vi "Change Output DT.vi"(6 "Variant":variant, 8 "error in (no error)":errorcluster, 9 "old values":string[][](array[string]), 10 "object ref in":T2, 11 "Cluster":T3) -> (0 "error out":errorcluster)   [LabVIEW 2013, in "Scaling editor node.lvclass"]
uses:
  Scaling editor node.lvclass
  <vilib>/NI/DCAF Table API/Table Manager/Cell Change.ctl
  <vilib>/NI/DCAF Table API/Table Manager/object ref.ctl
  <vilib>/NI/DCAF/Tag Editor Core/Configuration Editor/Classes/Engine Parent/Engine Parent Editor Node.lvclass
  <vilib>/NI/DCAF/Tag Editor Core/Configuration Editor/Classes/Module editor node/module editor node.lvclass
  module/configuration/controls/scale data types.ctl
  module/configuration/Scaling configuration.lvclass
  Scaling editor node.lvclass/Scaling editor node.ctl
  <vilib>/NI/DCAF Table API/Table Manager.lvlib
  <vilib>/NI/DCAF Table API/Table Manager/Table Manager.lvclass
panel:
  in  "dt":T1
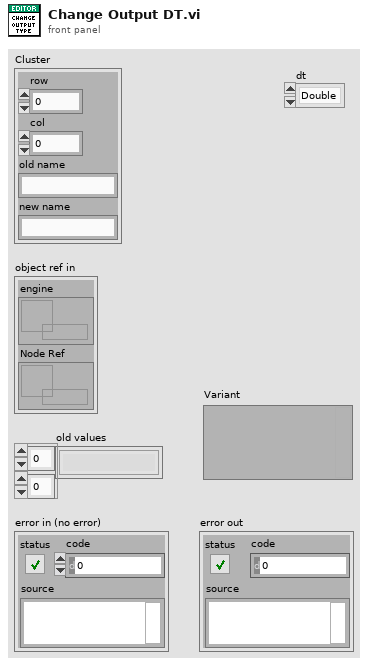
[diagram p1: front panel]
types:
  T1 = typedef "Scaling configuration.lvclass/scale data types.ctl" = enum16{"Double", "Single", "I64", "I32", "I16", "I8", "U64", "U32", "U16", "U8", "Boolean (0,1)"}
  T2 = typedef "Table Manager.lvlib/Table Manager.lvclass/object ref.ctl" = cluster{"engine":refnum<data-value>, "Node Ref":refnum<data-value>}
  T3 = typedef "Table Manager.lvlib/Cell Change.ctl" = cluster{"row":i32, "col":i32, "old name":string, "new name":string}
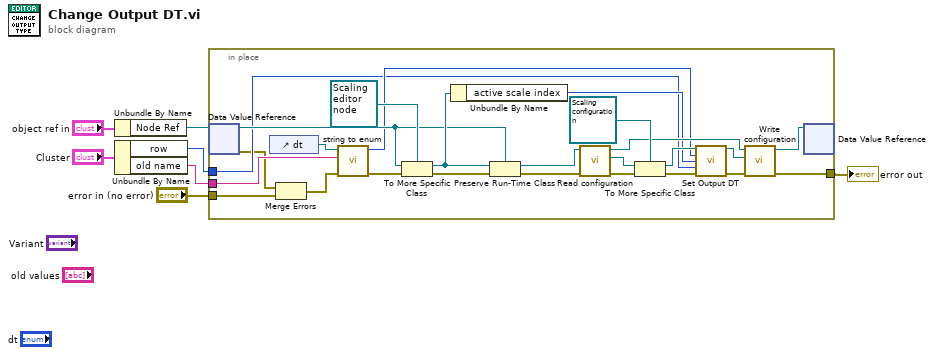
[diagram p0: block diagram]
diagram:
  n1 = Unbundle By Name("object ref in") -> ("Node Ref"=w3:refnum<data-value>)
  n2 = Unbundle By Name("Cluster") -> ("row"=w5:i32, "old name"=w2:string)
  n3 = in-place {
    in-place-border: w5 -> [w11]
    in-place-border: [w23] -> w1
    in-place-border: w2 -> [w14]
    in-place-border: "error in (no error)" -> [w9]
    n4 = in-place-dvr #1(w3) -> (w22:refnum<class "module editor node.lvclass">, w10:errorcluster)
    n5 = control-ref of="dt"() -> (w15:refnum<vi>)
    n6 = Merge Errors(w10, w9) -> (w8:errorcluster)
    n7 = call <vilib>:"string to enum.vi"("error in"=w8, "String"=w14, "Enum"=w15) -> ("error out"=w16:errorcluster, "Value"=w13:i32)  [unwired: 7 in]
    n8 = To More Specific Class(target class=refnum<class "Scaling editor node.lvclass"> refnum ("Scaling editor node"), reference=w22, error in=w16) -> (specific class reference=w28:refnum<class "Scaling editor node.lvclass">, error out=w21:errorcluster)
    n9 = Unbundle By Name(w28) -> ("active scale index"=w12:i32)
    n10 = Preserve Run-Time Class(object in=w28, error in=w21, 2:w22) -> (object out=w27:refnum<class "module editor node.lvclass">, error out=w26:errorcluster)
    n11 = call-dynamic "Read configuration.vi"("error in"=w26, "NISE_CEF_serializable node in"=w27) -> ("error out"=w25:errorcluster, "configuration"=w30:refnum<class "NISE_CEF_serializable configuration.lvclass">, "NISE_CEF_serializable node out"=w24:refnum<class "module editor node.lvclass">)  [unwired: 7 in]
    n12 = To More Specific Class(target class=refnum<class "Scaling configuration.lvclass"> refnum ("Scaling configuration"), reference=w30, error in=w25) -> (specific class reference=w17:refnum<class "Scaling configuration.lvclass">, error out=w18:errorcluster)
    n13 = call "Set Output DT.vi"("Scaling configuration in"=w17, "Scale Data Type"=w13, "Scale Index"=w12, "Mapping Index"=w11, "error in (no error)"=w18) -> ("Scaling configuration out"=w20:refnum<class "Scaling configuration.lvclass">, "error out"=w19:errorcluster)  [unwired: 9 in]
    n14 = call-dynamic "Write configuration.vi"("error in"=w19, "configuration"=w20, "NISE_CEF_serializable node in"=w24) -> ("error out"=w23:errorcluster, "NISE_CEF_serializable node out"=w32:refnum<class "module editor node.lvclass">)  [unwired: 7 in]
    n15 = in-place-dvr #1(w32) -> ()  [unwired: 2 out]
  }
  "error out" <- w1
